vi "Get Params.vi"(1 "USAC Params in":refnum<class "USAC Params.lvclass">) -> (0 "Parameters":T1)   [LabVIEW 2020, in "g_ar_toolkit.ar.lvlib" / "USAC Params.lvclass"]
uses:
  USAC Params.lvclass
  USAC Params.lvclass/USAC Params.ctl
  Polishing Methods.ctl
  Local Optimization Methods.ctl
  Neighbor Search Methods.ctl
  Sampling Methods.ctl
  Score Methods.ctl
  Parameters.ctl
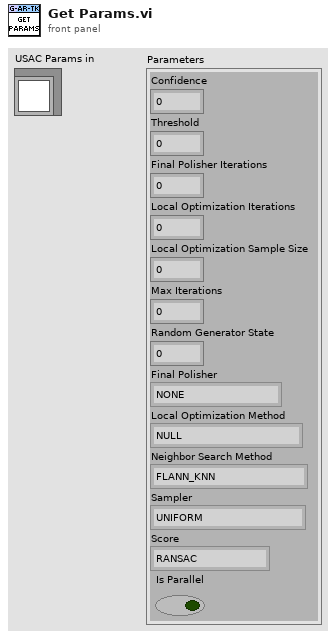
[diagram p1: front panel]
types:
  T1 = typedef "g_ar_toolkit.ar.lvlib/USAC Params.lvclass/Parameters.ctl" = cluster{"Confidence":dbl, "Threshold":dbl, "Final Polisher Iterations":i32, "Local Optimization Iterations":u16, "Local Optimization Sample Size":u16, "Max Iterations":u16, "Random Generator State":i32, "Final Polisher":T2, "Local Optimization Method":T3, "Neighbor Search Method":T4, "Sampler":T5, "Score":T6, "Is Parallel":bool}
  T2 = typedef "g_ar_toolkit.ar.lvlib/USAC Params.lvclass/Polishing Methods.ctl" = enum8{"NONE", "LSQ", "MAGSAC", "COV"}
  T3 = typedef "g_ar_toolkit.ar.lvlib/USAC Params.lvclass/Local Optimization Methods.ctl" = enum8{"NULL", "INNER_LO", "INNER_AND_ITER_LO", "GC", "SIGMA"}
  T4 = typedef "g_ar_toolkit.ar.lvlib/USAC Params.lvclass/Neighbor Search Methods.ctl" = enum8{"FLANN_KNN", "GRID", "FLANN_RADIUS"}
  T5 = typedef "g_ar_toolkit.ar.lvlib/USAC Params.lvclass/Sampling Methods.ctl" = enum8{"UNIFORM", "PROGRESSIVE_NAPSAC", "NAPSAC", "PROSAC"}
  T6 = typedef "g_ar_toolkit.ar.lvlib/USAC Params.lvclass/Score Methods.ctl" = enum8{"RANSAC", "MSAC", "MAGSAC", "LMEDS"}
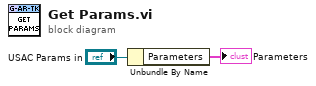
[diagram p0: block diagram]
diagram:
  n1 = Unbundle By Name("USAC Params in") -> ("Parameters"=→"Parameters":T1)
